vi "Inverse Filter Demo-3.vi"() -> ()   [LabVIEW 2015]
uses:
  Calibration VIs/Inverse Filter VIs/InvFilt-Params.ctl
  <vilib>/Analysis/4window.llb/Modified Bartlett-Hanning Window (DBL).vi
  Utility VIs/Math VIs/FFT x(t) to dB,Degrees (1D).vi
  Utility VIs/Math VIs/Linear to dB (array).vi
  <vilib>/Analysis/NI_AALPro.lvlib
panel:
  in  "InvFilt Params":T1={"Min Frequency (Hz)"=1000.0, "Max Frequency (Hz)"=100000.0, "Length (points)"=1000000, "Sampling rate (Hz)"=100000.0, "Delay (ms)"=1.5, "Linear phase"=FALSE}
  in  "T (s)":dbl=0.5
  in  "Fs (Hz)":dbl=100000.0
  out "Noise out":cluster{"Frequency (Hz)":dbl[], "dB":dbl[]}[](graph)
  in  "Calibration file":path=path "C:/Experiment VIs/Signal Generation VIs/Test VIs/RightPrimary.calib"
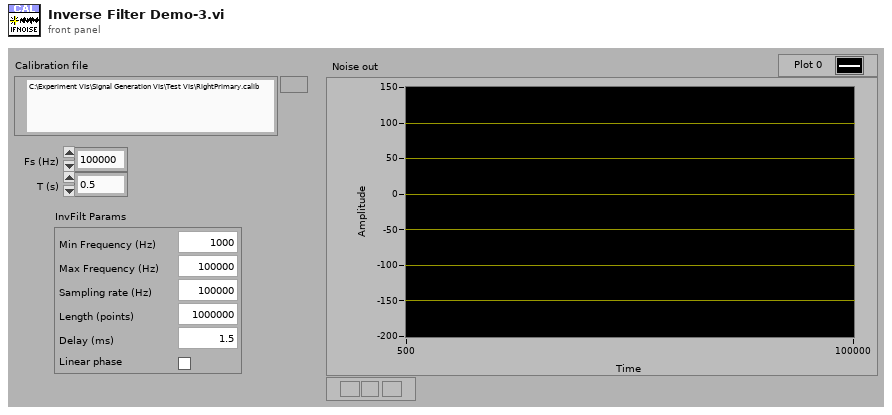
[diagram p1: front panel]
types:
  T1 = typedef "InvFilt-Params.ctl" = cluster{"Min Frequency (Hz)":dbl, "Max Frequency (Hz)":dbl, "Length (points)":i32, "Sampling rate (Hz)":dbl, "Delay (ms)":dbl, "Linear phase":bool}
  T2 = cluster{"Interp Freq (Hz)":dbl[], "Interp Magnitude (dB)":dbl[]}
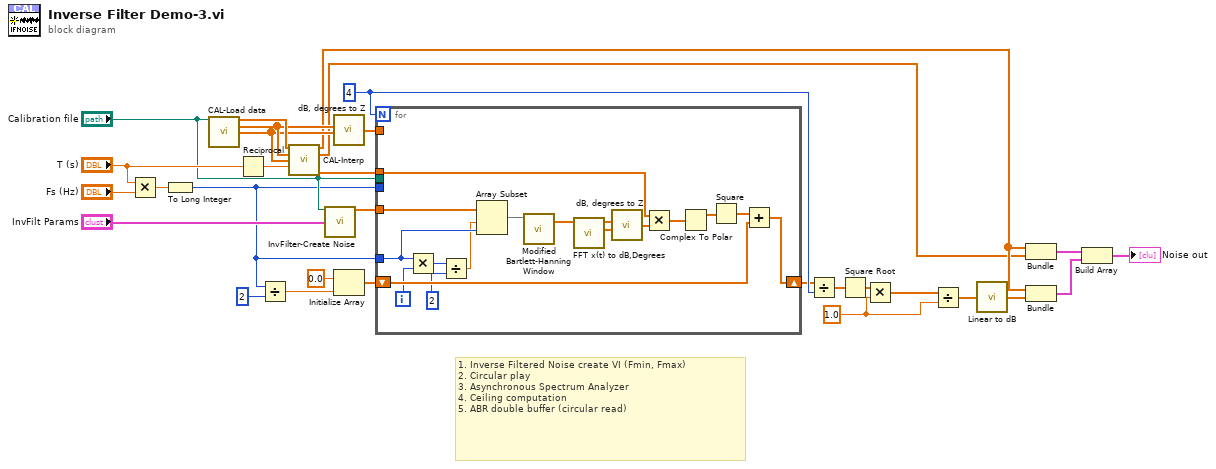
[diagram p0: block diagram]
diagram:
  w2 = 1.0
  w27 = 4
  # "1. Inverse Filtered Noise create VI (Fmin, Fmax)\n2. Circular play\n3. Asynchronous Spectrum Analyzer\n4. Ceiling computation\n5. ABR double buffer (circular read)"
  n1 = Multiply(x="T (s)", y="Fs (Hz)") -> (x*y=w23:dbl)
  n2 = To Long Integer(number=w23) -> (32bit integer=w6:i32)
  n3 = call "CAL-Load data.vi"("user path"="Calibration file") -> ("Frequency (Hz)"=w20:dbl[], "Mag"=w19:dbl[], "Phase"=w18:dbl[])  [unwired: 7 in, 5 out]
  n4 = Reciprocal(x="T (s)") -> (1/x=w17:dbl)
  n5 = Divide(x=w6, y=2) -> (x/y=w7:dbl)
  n6 = call "CAL-Interp.vi"("Frequency (Hz)"=w20, "Magnitude (dB)"=w19, "Phase (degrees)"=w18, "df (Hz)"=w17) -> ("Interp Freq (Hz)"=w15:dbl[], "Interp Magnitude (dB)"=w9:dbl[], "Interp z"=w14:cdb[])  [unwired: 8 in, 1 out]
  n7 = call "InvFilter-Create Noise.vi"("Calibration File"="Calibration file", "InvFilt Params"="InvFilt Params") -> ("InvFilter Noise"=w1:dbl[])  [unwired: 10 in, 3 out]
  n8 = call "dB, degrees to Z.vi"("Magnitude (dB)"=w19, "Phase (degrees)"=w18) -> ("Z"=w30:cdb[])  [unwired: 5 in]
  n9 = Initialize Array(0.0 ("element"), w7) -> (w29:dbl[])
  n10 = for {
    N: w27 -> [_]
    tunnel: w30 -> [_]
    shift-right: [w46] -> w4
    shift-left: w29 -> [w45]
    tunnel: w6 -> [_]
    tunnel: w14 -> [w43]
    tunnel: "Calibration file" -> [_]
    tunnel: w1 -> [w42]
    tunnel: w6 -> [w39]
    i -> [w41]
    n11 = Multiply(x=w39, y=w41) -> (x*y=w40:i32)
    n12 = Divide(x=w40, y=2) -> (x/y=w38:dbl)
    n13 = Array Subset(array=w42, index=w38, length=w39) -> (w34:dbl[])
    n14 = call-poly <vilib>:"Modified Bartlett-Hanning Window.vi"("X"=w34) -> ("Windowed X"=w33:dbl[])  [unwired: 9 in, 1 out]
    n15 = call-poly "FFT x(t) to dB,Degrees.vi"("X"=w33) -> ("+Freq Phase of FFT (degrees)"=w47:dbl[], "+Freq. Mag of FFT (dB rms)"=w44:dbl[])  [unwired: 8 in, 1 out]
    n16 = call "dB, degrees to Z.vi"("Magnitude (dB)"=w44, "Phase (degrees)"=w47) -> ("Z"=w32:cdb[])  [unwired: 5 in]
    n17 = Multiply(x=w43, y=w32) -> (x*y=w31:cdb[])
    n18 = Complex To Polar(r * e^(i*theta)=w31) -> (r=w36:dbl[])  [unwired: 1 out]
    n19 = Square(x=w36) -> (x^2=w35:dbl[])
    n20 = Add(x=w35, y=w45) -> (x+y=w46:dbl[])
  }
  n21 = Divide(x=w4, y=w27) -> (x/y=w10:dbl[])
  n22 = Square Root(x=w10) -> (sqrt(x)=w3:dbl[])
  n23 = Multiply(x=w3, y=w2) -> (x*y=w8:dbl[])
  n24 = Divide(x=w8, y=w2) -> (x/y=w5:dbl[])
  n25 = call-poly "Linear to dB.vi"("linear"=w5) -> ("dB"=w11:dbl[])
  n26 = Bundle("Interp Freq (Hz)"=w15, "Interp Magnitude (dB)"=w9) -> (w24:T2)  [unwired: 1 in]
  n27 = Bundle("Interp Freq (Hz)"=w15, "dB"=w11) -> (w26:cluster{"Interp Freq (Hz)":dbl[], "dB":dbl[]})  [unwired: 1 in]
  n28 = Build Array(w24, w26) -> (→"Noise out":cluster{"Interp Freq (Hz)":dbl[], "dB":dbl[]}[])
